vi "Configure Trigger (Communication - AMI Or Subtypes).vi"(0 "VISA resource name":refnum<visa-resource-name>, 1 "Coding (2:AMI)":u16(ring)=2 items=["AMI"=2, "HDB3"=3, "B3ZS"=4, "B6ZS"=5, "B8ZS"=6], 2 "Standard (3:Clock Coax)":u16(ring)=3 items=["Clock Coax"=3, "Clock Symmetrical"=4, "DS0 Contra"=7, "DS0 Double"=8, "DS0 Single"=9, "DS0Timing"=10, "DS1"=11, "DS1A"=12, "DS1C"=13, "DS2"=14, "DS2RATE Symmetrical"=15, "DS2RATE Coax"=16, "RATE32Mbit"=17, "RATE97Mbit"=18, "DS3"=19, "E1"=21, "E2"=22, "E3"=23, "STM0_HDBX"=59, "Custom"=70], 3 "Bit Rate (1.544Mb/s)":dbl=1544000.0, 5 "Source (0:Channel1)":u16(ring) items=["Channel1", "Channel2", "Channel3", "Channel4"], 7 "Source Type (0:Data)":u16(ring) items=["Data", "Clock", "Recovered"], 9 "Pulse Form (0: 1)":u16(ring) items=["+1", "-1", "Eye"], 11 "error in (no error)":errorcluster, 12 "Data Type":T1={"Upper Level (1.2V)"=1.2, "Lower Level (0.8V)"=0.8}, 13 "Clock Type":T2 {"Clock Polarity (0:Positive)" items=["Positive", "Negative"]}) -> (4 "VISA resource name out":refnum<visa-resource-name>, 15 "error out":errorcluster)   [LabVIEW 2012, in "Tektronix 7000 Series.lvlib"]
doc: "Configures Communication trigger settings for an oscilloscope.A trigger occurs when a communications signal is found. Supports AMI,HDB3,B3ZS,B6ZS and B8ZS encoded communications signals.\n\nTDS5000,TDS5000B series oscilloscopes don't support this trigger."
uses:
  Tektronix 7000 Series.lvlib
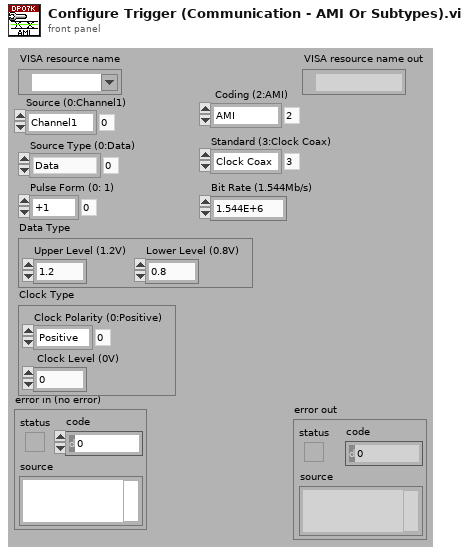
[diagram p1: front panel]
types:
  T1 = cluster{"Upper Level (1.2V)":dbl, "Lower Level (0.8V)":dbl}
  T2 = cluster{" Clock Level (0V)":dbl, "Clock Polarity (0:Positive)":u16}
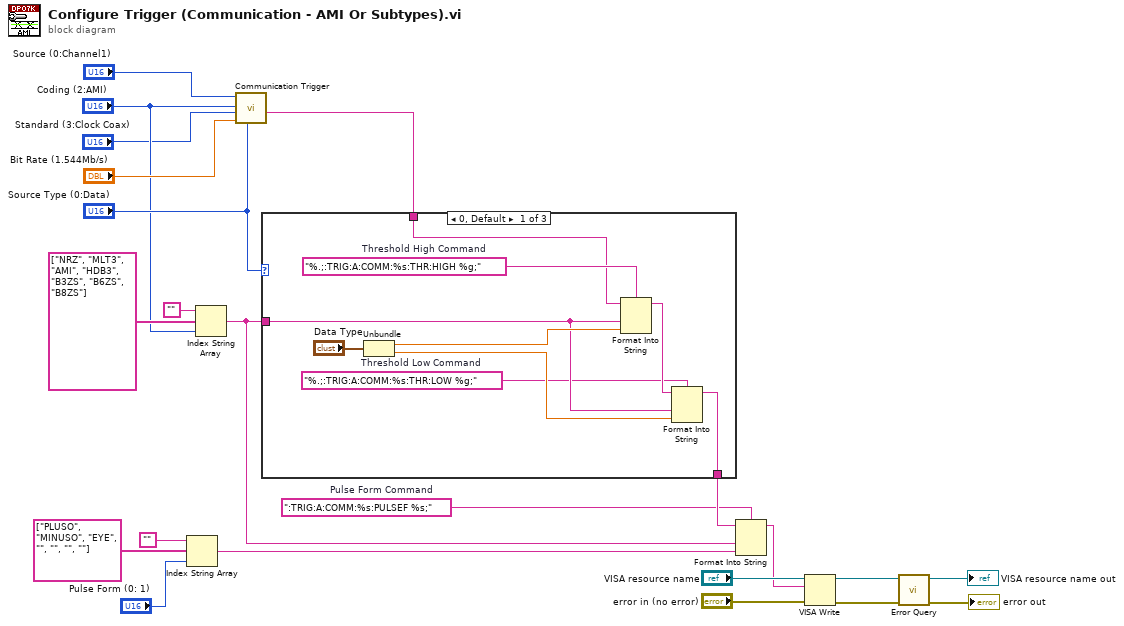
[diagram p0: block diagram]
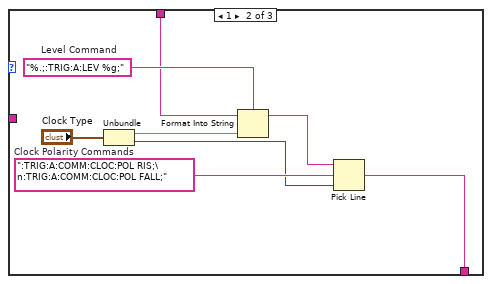
[diagram p2: hidden frame]
diagram:
  w9 = ":TRIG:A:COMM:%s:PULSEF %s;"  # Pulse Form Command
  n1 = Index String Array(1:"Pulse Form (0: 1)", 2:string[] ["PLUSO", "MINUSO", "EYE", "", "", "", ""], 3:"") -> (0:w10:string)
  n2 = Index String Array(1:"Coding (2:AMI)", 2:string[] ["NRZ", "MLT3", "AMI", "HDB3", "B3ZS", "B6ZS", "B8ZS"], 3:"") -> (0:w14:string)
  n3 = call "Communication Trigger.vi"("Source Type (0:Data)"="Source Type (0:Data)", "Bit Rate (1.544E6Mb/s)"="Bit Rate (1.544Mb/s)", "Standard (0:ATAG1)"="Standard (3:Clock Coax)", "Coding (0:NRZ)"="Coding (2:AMI)", "Source (0:Channel1)"="Source (0:Channel1)") -> ("Output String"=w19:string)  [unwired: 6 in]
  n4 = case shown="0, Default" "Source Type (0:Data)" {
    tunnel: w19 -> [w28 w37 w40]
    tunnel: w14 -> [w25 _ _]
    tunnel: [w23 w32 w40] -> w15
    frame 0, Default {
      w24 = "%.;:TRIG:A:COMM:%s:THR:LOW %g;"  # Threshold Low Command
      w29 = "%.;:TRIG:A:COMM:%s:THR:HIGH %g;"  # Threshold High Command
      n5 = Unbundle("Data Type") -> ("Upper Level (1.2V)"=w30:dbl, "Lower Level (0.8V)"=w26:dbl)
      n6 = Format Into String(format string=w29, initial string=w28, w25, w30) -> (resulting string=w27:string)  [unwired: 1 in, 1 out]
      n7 = Format Into String(format string=w24, initial string=w27, w25, w26) -> (resulting string=w23:string)  [unwired: 1 in, 1 out]
    }
    frame 1 {
      w34 = ":TRIG:A:COMM:CLOC:POL RIS;\n:TRIG:A:COMM:CLOC:POL FALL;"  # Clock Polarity Commands
      w38 = "%.;:TRIG:A:LEV %g;"  # Level Command
      n8 = Unbundle("Clock Type") -> ("Clock Level (0V)"=w36:dbl, "Clock Polarity (0:Positive)"=w33:u16)
      n9 = Format Into String(format string=w38, initial string=w37, w36) -> (resulting string=w35:string)  [unwired: 1 in, 1 out]
      n10 = Pick Line(string ("")=w35, multi-line string=w34, line index=w33) -> (output string=w32:string)
    }
    frame 2 {
    }
  }
  n11 = Format Into String(format string=w9, initial string=w15, w14, w10) -> (resulting string=w2:string)  [unwired: 1 in, 1 out]
  n12 = VISA Write(VISA resource name="VISA resource name", write buffer=w2, error in (no error)="error in (no error)") -> (VISA resource name out=w8:refnum<visa-resource-name>, error out=w7:errorcluster)  [unwired: 1 out]
  n13 = call "Error Query.vi"("error in (no error)"=w7, "VISA resource name"=w8) -> ("error out"=→"error out":errorcluster, "VISA resource name out"=→"VISA resource name out":refnum<visa-resource-name>)  [unwired: 6 in, 2 out]
